vi "Colour Row.vi"(6 "Row Colour":u32, 7 "MulticolumnListbox in":refnum<vi>, 8 "error in (no error)":errorcluster, 10 "Row Number":i32) -> (0 "error out":errorcluster)   [LabVIEW 2016, in "Assert API Components.lvlib" / "Assert Display.lvlib" / "Main Display.lvlib" / "Main Display.lvclass"]
doc: "Applies a specified colour to every cell that is visible in a selected row."
uses:
  Main Display.lvclass
  <vilib>/Utility/miscctls.llb/LVRowAndColumnTypeDef.ctl
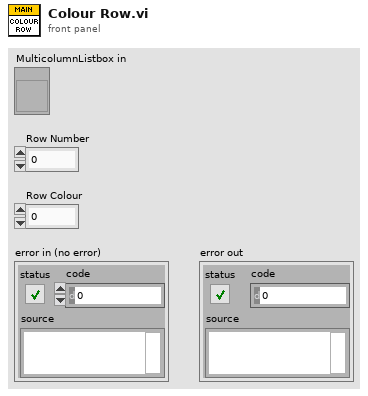
[diagram p1: front panel]
types:
  T1 = typedef "LVRowAndColumnTypeDef.ctl" = cluster{"Row":i32, "Column":i32}
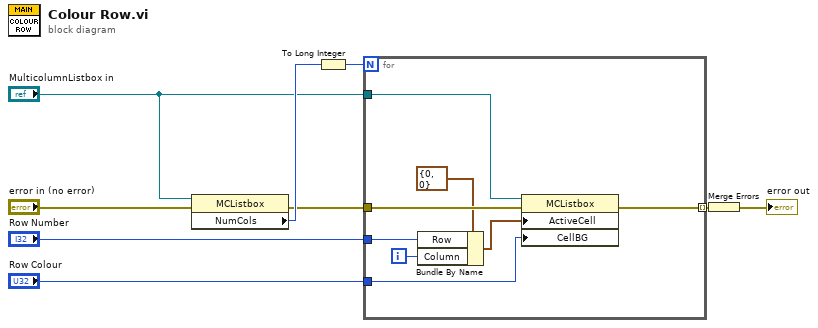
[diagram p0: block diagram]
diagram:
  n1 = property class="MCListbox"(reference="MulticolumnListbox in", error in="error in (no error)") -> (error out=w5:errorcluster, "NumCols"=w7:u32)  [unwired: 1 out]
  n2 = To Long Integer(number=w7) -> (32bit integer=w8:i32)
  n3 = for {
    N: w8 -> [_]
    tunnel: "MulticolumnListbox in" -> [w15]
    tunnel: "Row Number" -> [w12]
    tunnel: "Row Colour" -> [w10]
    tunnel: w5 -> [w17]
    tunnel: [w16] -> w3 mode=indexing
    i -> [w13]
    n4 = Bundle By Name(cluster=T1 {"Row"=0, "Column"=0} ("Active Cell:Active Cell"), "Row"=w12, "Column"=w13) -> (w14:T1)
    n5 = property class="MCListbox"(reference=w15, error in=w17, "ActiveCell"=w14, "CellBG"=w10) -> (error out=w16:errorcluster)  [unwired: 1 out]
  }
  n6 = Merge Errors(w3) -> (→"error out":errorcluster)
